vi "Test zmq.vi"() -> ()   [LabVIEW 2019, in "Communication Interface.lvlib"]
uses:
  Communication Interface.lvlib
  <vilib>/addons/zeromq/socket_type.ctl
  <vilib>/Analysis/1siggen.llb/Ramp Pattern by Samples.vi
  <vilib>/addons/zeromq/zmq_context.lvclass
  <vilib>/addons/zeromq/zeromq.lvlib
  <vilib>/addons/zeromq/zmq_socket.lvclass
  <vilib>/Analysis/NI_AALBase.lvlib
panel:
  out "resp":string
  out "status":string
  in  "plot":bool
  out "duraiton":dbl format="%#_6p"
  in  "samples":i32=3200000
  in  "Start command":string="{\t    \"Bursts\":[\t        \"Chrip_250MHz\"\t    ],\t    \"Acquisition length\":320000\t}"
  out "iq data":sgl[][](graph)
  in  "command":string(combo)
  in  "send":bool
  out "attempt":i32
  in  "stop":bool
  in  "ntries":i32=1
  in  "endpoint":string="tcp://127.0.0.1:5555"
  in  "timeout":u32=1000
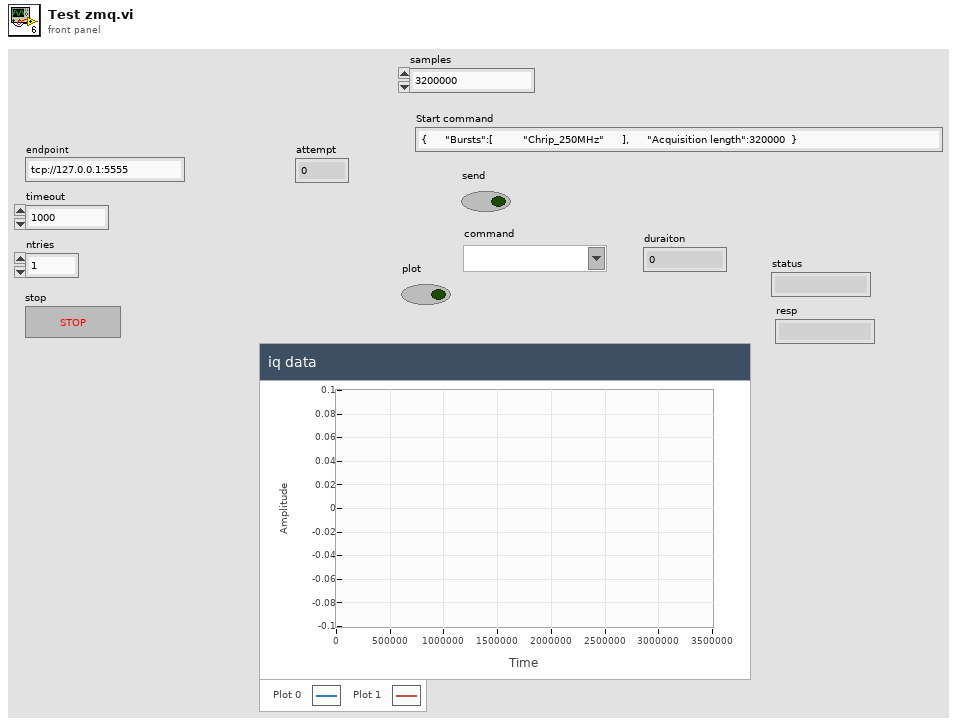
[diagram p1: front panel]
types:
  T1 = typedef "zeromq.lvlib/socket_type.ctl" = enum8{"ZMQ_PAIR", "ZMQ_PUB", "ZMQ_SUB", "ZMQ_REQ", "ZMQ_REP", "ZMQ_DEALER", "ZMQ_ROUTER", "ZMQ_PULL", "ZMQ_PUSH", "ZMQ_XPUB", "ZMQ_XSUB"}
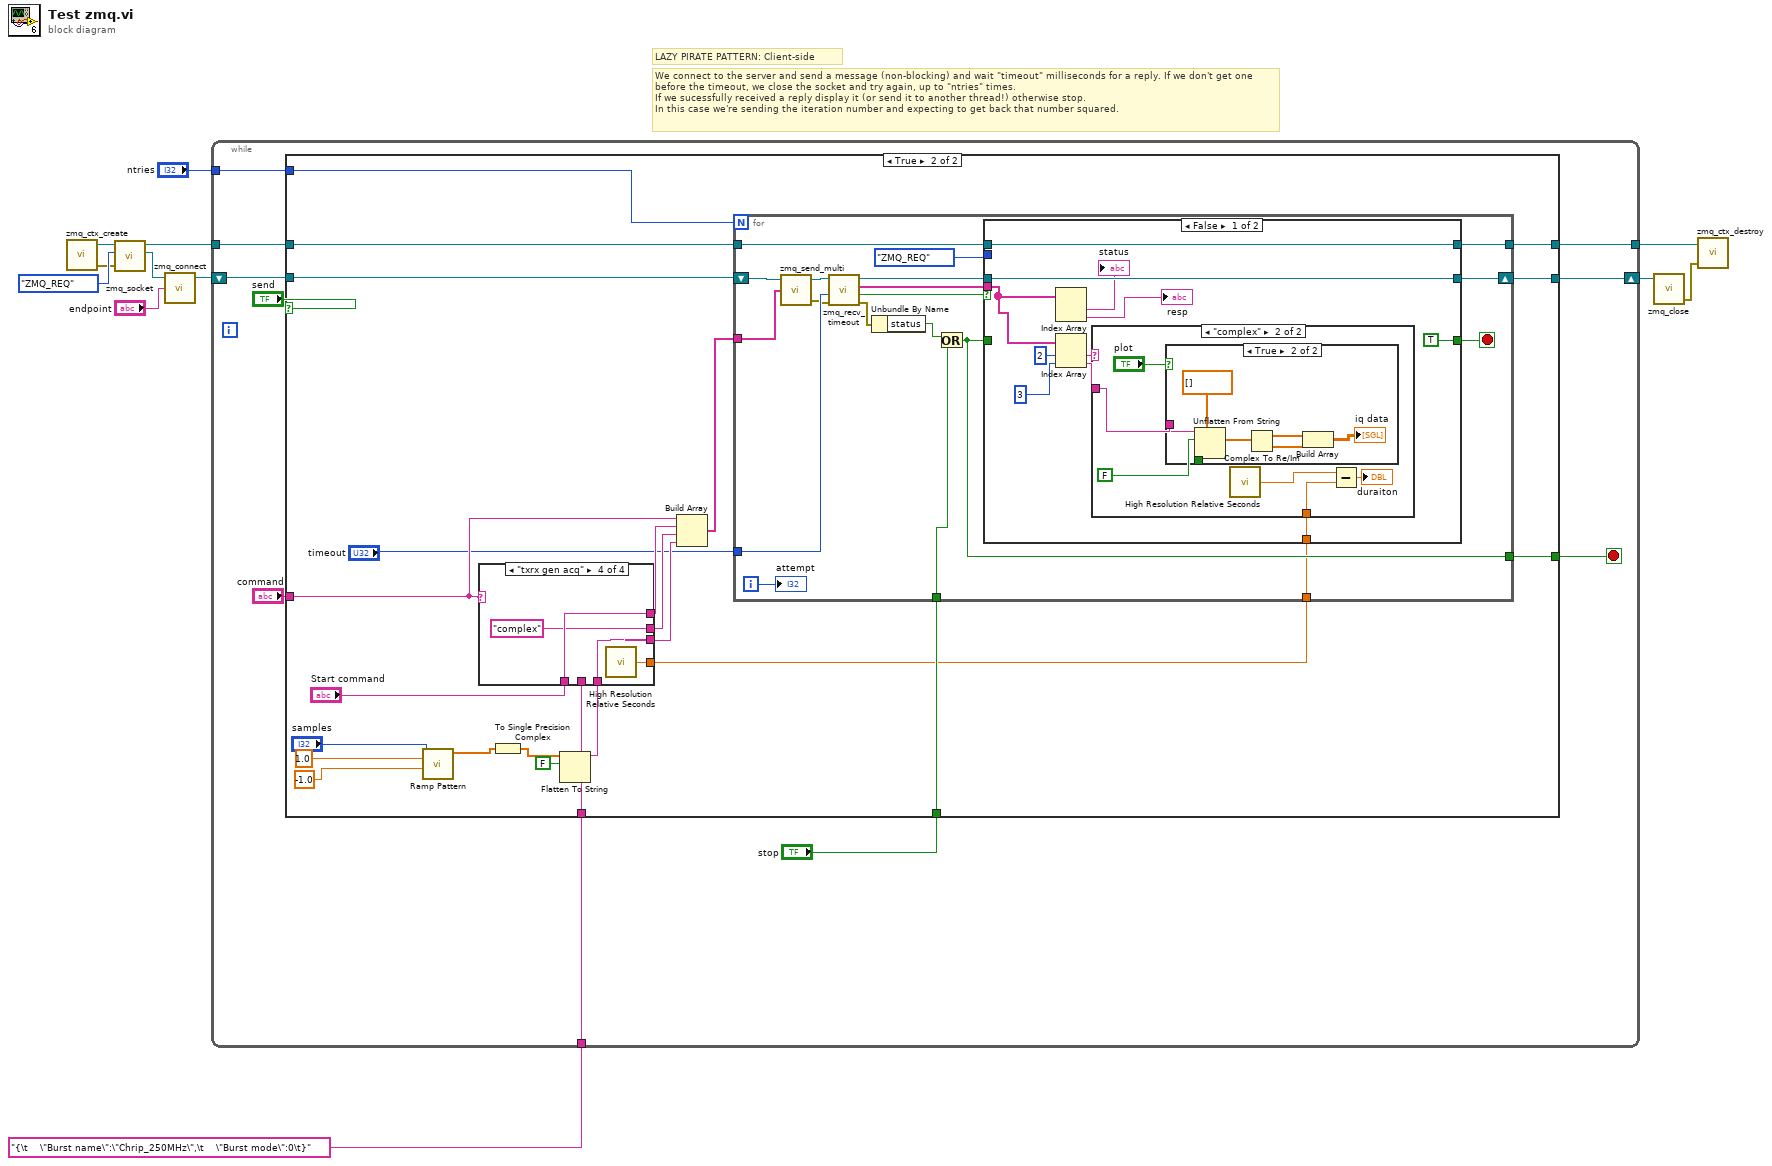
[diagram p0: block diagram]
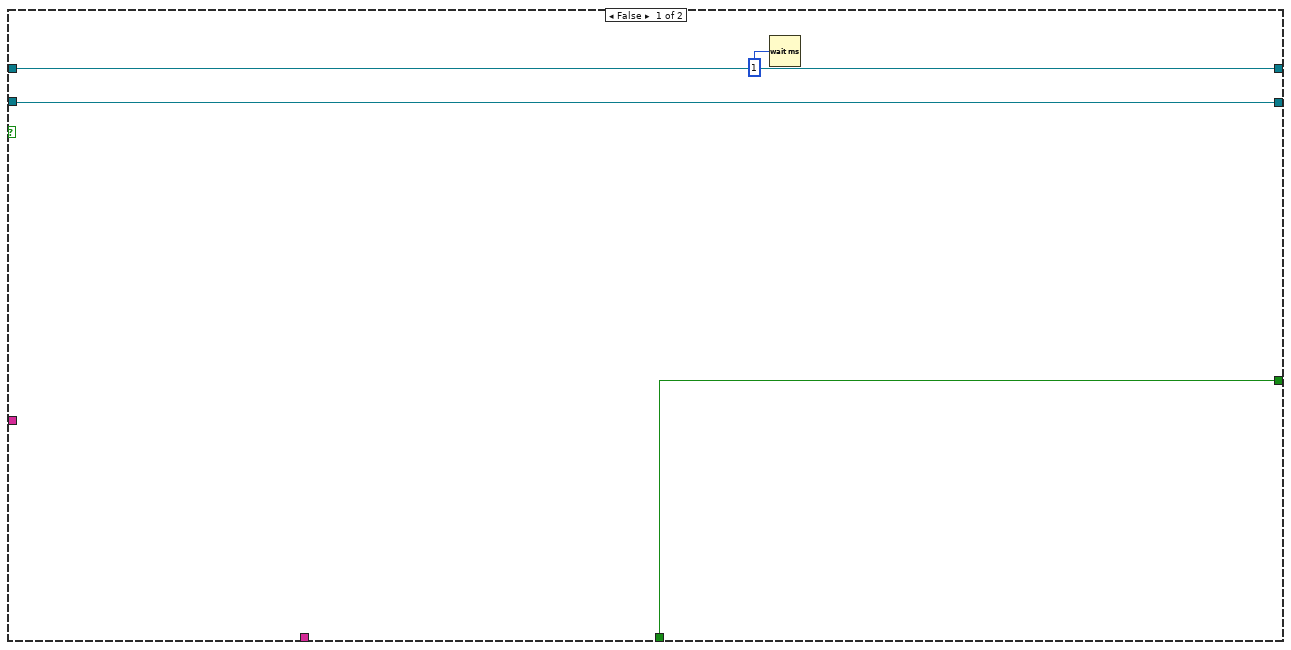
[diagram p2: hidden frame]
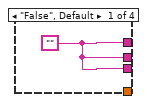
[diagram p3: hidden frame]
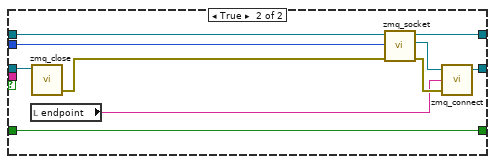
[diagram p8: hidden frame]
diagram:
  # "We connect to the server and send a message (non-blocking) and wait \"timeout\" milliseconds for a reply. If we don't get one before the timeout, we close the socket and try again, up to \"ntries\" times.\nIf we sucessfully received a reply display it (or send it to another thread!) otherwise stop.\nIn this case we're sending the iteration number and expecting to get back that number squared."
  # "LAZY PIRATE PATTERN: Client-side"
  n1 = call <vilib>:"zmq_ctx_create.vi"() -> ("error out"=w2:errorcluster, "context out"=w11:refnum<class "zmq_context.lvclass">)  [unwired: 4 in]
  n2 = call <vilib>:"zmq_socket.vi"("error in"=w2, "socket type"=socket_type."ZMQ_REQ", "context in"=w11) -> ("socket out"=w9:refnum<class "zmq_socket.lvclass">, "context out"=w8:refnum<class "zmq_context.lvclass">)  [unwired: 2 in, 1 out]
  n3 = call <vilib>:"zmq_connect.vi"("endpoint"="endpoint", "socket in"=w9) -> ("socket out"=w6:refnum<class "zmq_socket.lvclass">)  [unwired: 2 in, 1 out]
  n4 = while {
    tunnel: w8 -> [w22]
    tunnel: "ntries" -> [w21]
    tunnel: [w19] -> w5
    shift-right: [w18] -> w4
    shift-left: w6 -> [w20]
    tunnel: "{\t    \"Burst name\":\"Chrip_250MHz\",\t    \"Burst mode\":0\t}" -> [w14]
    stop <- w13 stop-if-true
    n5 = case shown="True" "send" {
      tunnel: w22 -> [w26 w49]
      tunnel: w21 -> [_ w48]
      tunnel: [w24 w47] -> w13
      tunnel: w20 -> [w25 w46]
      tunnel: [w26 w45] -> w19
      tunnel: [w25 w44] -> w18
      tunnel: "stop" -> [w24 w43]
      tunnel: "command" -> [_ w41]
      tunnel: w14 -> [_ w39]
      frame False {
        n6 = Wait (ms)(milliseconds to wait=u32 1) -> ()  [unwired: 1 out]
      }
      frame True {
        n7 = call-poly <vilib>:"Ramp Pattern.vi"("start"=-1.0, "end"=1.0 ("start"), "samples"="samples") -> ("Ramp Pattern"=w33:dbl[])  [unwired: 7 in, 1 out]
        n8 = To Single Precision Complex(1:w33) -> (0:w34:csg[])
        n9 = Flatten To String(anything=w34, prepend array or string size? (T)=FALSE) -> (data string=w29:string)  [unwired: 2 in, 2 out]
        n10 = case shown="\"txrx gen acq\"" w41 {
          tunnel: [w50 w51 w52 w56] -> w40
          tunnel: "Start command" -> [_ w51 _ w56]
          tunnel: w39 -> [_ _ w52 _]
          tunnel: [w50 _ _ "complex"] -> w38
          tunnel: [w50 _ _ w54] -> w37
          tunnel: w29 -> [_ _ _ w54]
          tunnel: [_ _ _ w53] -> w28
          frame "False", Default {
            w50 = ""
          }
          frame "start" {
          }
          frame "trigger burst" {
          }
          frame "txrx gen acq" {
            n11 = call <vilib>:"High Resolution Relative Seconds.vi"() -> ("relative seconds"=w53:dbl)
          }
        }
        n12 = Build Array(w41, w40, w38, w37) -> (w42:string[])
        n13 = for {
          N: w48 -> [_]
          tunnel: w49 -> [w63]
          tunnel: "timeout" -> [w74]
          tunnel: w42 -> [w58]
          tunnel: [w66] -> w47
          shift-right: [w62] -> w44
          shift-left: w46 -> [w64]
          tunnel: [w61] -> w45
          tunnel: w43 -> [w59]
          tunnel: w28 -> [w57]
          i -> [w70]
          stop <- w65 stop-if-true
          n14 = call <vilib>:"zmq_send_multi.vi"("parts"=w58, "socket in"=w64) -> ("error out"=w71:errorcluster, "socket out"=w72:refnum<class "zmq_socket.lvclass">)  [unwired: 2 in]
          n15 = call <vilib>:"zmq_recv_timeout.vi"("error in"=w71, "timeout (ms)"=w74, "socket in"=w72) -> ("error out"=w69:errorcluster, "timeout?"=w68:bool, "parts"=w73:string[], "socket out"=w75:refnum<class "zmq_socket.lvclass">)  [unwired: 1 in]
          n16 = Unbundle By Name(w69) -> ("status"=w67:bool)
          n17 = Or(x=w67, y=w59) -> (x .or. y?=w66:bool)
          n18 = case shown="False" w68 {
            tunnel: w75 -> [w85 w109]
            tunnel: w73 -> [w78 _]
            tunnel: w66 -> [_ w108]
            tunnel: [TRUE w108] -> w65
            tunnel: w63 -> [w84 w107]
            tunnel: [w85 w102] -> w62
            tunnel: [w84 w104] -> w61
            tunnel: socket_type."ZMQ_REQ" ("socket type") -> [_ w101]
            tunnel: w57 -> [w79 _]
            frame False {
              n19 = Index Array(array=w78) -> (element #1=→"status":string, element #2=→"resp":string)  [unwired: 2 in]
              n20 = Index Array(array=w78, index #1=2 ("index"), index #2=3 ("index")) -> (element #1=w81:string, element #2=w80:string)
              n21 = case shown="\"complex\"" w81 {
                tunnel: w80 -> [_ w91]
                tunnel: w79 -> [_ w90]
                frame "False", Default {
                }
                frame "complex" {
                  n22 = case shown="True" "plot" {
                    tunnel: FALSE -> [_ w98]
                    tunnel: w91 -> [_ w93]
                    frame False {
                    }
                    frame True {
                      n23 = Unflatten From String(type=csg[] [], binary string=w93, data includes array or string size? (T)=w98) -> (value=w97:csg[])  [unwired: 2 in, 2 out]
                      n24 = Complex To Re/Im(x + iy=w97) -> (x=w96:sgl[], y=w94:sgl[])
                      n25 = Build Array(w96, w94) -> (→"iq data":sgl[][])
                    }
                  }
                  n26 = call <vilib>:"High Resolution Relative Seconds.vi"() -> ("relative seconds"=w89:dbl)
                  n27 = Subtract(x=w89, y=w90) -> (x-y=→"duraiton":dbl)
                }
              }
            }
            frame True {
              n28 = local read "endpoint"() -> (w100:string)
              n29 = call <vilib>:"zmq_close.vi"("socket"=w109) -> ("error out"=w106:errorcluster)  [unwired: 4 in]
              n30 = call <vilib>:"zmq_socket.vi"("error in"=w106, "socket type"=w101, "context in"=w107) -> ("error out"=w105:errorcluster, "socket out"=w103:refnum<class "zmq_socket.lvclass">, "context out"=w104:refnum<class "zmq_context.lvclass">)  [unwired: 2 in]
              n31 = call <vilib>:"zmq_connect.vi"("error in"=w105, "endpoint"=w100, "socket in"=w103) -> ("socket out"=w102:refnum<class "zmq_socket.lvclass">)  [unwired: 1 in, 1 out]
            }
          }
          "attempt" <- w70
        }
      }
    }
  }
  n32 = call <vilib>:"zmq_close.vi"("socket"=w4) -> ("error out"=w3:errorcluster)  [unwired: 4 in]
  n33 = call <vilib>:"zmq_ctx_destroy.vi"("error in"=w3, "context in"=w5) -> ()  [unwired: 3 in, 1 out]
